vi "5s time subvi.vi"(10 "Main wash TimeElapsed":dbl, 11 "Main wash":dbl) -> (2 "Numeric":dbl, 3 "Numeric 2":dbl)   [LabVIEW 2019]
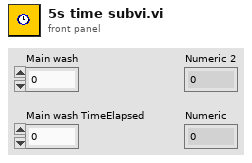
[diagram p1: front panel]
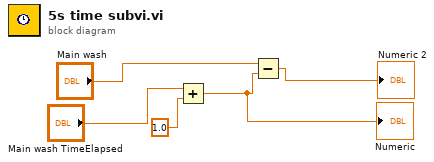
[diagram p0: block diagram]
diagram:
  n1 = Add(x="Main wash TimeElapsed", y=1.0) -> (x+y=w3:dbl)
  "Numeric" <- w3
  n2 = Subtract(x="Main wash", y=w3) -> (x-y=→"Numeric 2":dbl)
